vi "Top Level.vi"() -> ()   [LabVIEW 2018]
uses:
  Controls/DDS State.ctl
  <vilib>/ORNL/CSEISMIC DDS/CSEISMIC DDS Base/CSEISMIC DDS.lvclass/CSEISMIC DDS.ctl
  <vilib>/ORNL/CSEISMIC DDS/DDS Writer/Initializers/Initialize IED_Status_0 Writer.vi
  <vilib>/ORNL/CSEISMIC DDS/DDS Reader/Initializers/Initialize IED_setMicrogridID Reader.vi
  <vilib>/ORNL/CSEISMIC DDS/DDS Reader/Initializers/Initialize DER_Control Reader.vi
  <vilib>/ORNL/CSEISMIC DDS/DDS Reader/Initializers/Initialize DER_setPointP Reader.vi
  <vilib>/ORNL/CSEISMIC DDS/DDS Reader/Initializers/Initialize DER_SetPointQ Reader.vi
  <vilib>/ORNL/CSEISMIC DDS/DDS Reader/Initializers/Initialize IED_watchdogReset Reader.vi
  <vilib>/ORNL/CSEISMIC DDS/DDS Writer/Initializers/Initialize DER_Info Writer.vi
  <vilib>/ORNL/CSEISMIC DDS/DDS Writer/Initializers/Initialize DER_Measurement Writer.vi
  <vilib>/ORNL/CSEISMIC DDS/DDS Writer/Initializers/Initialize DER_Status Writer.vi
  <vilib>/ORNL/CSEISMIC DDS/DDS Writer/Initializers/Initialize IED_Status Writer.vi
  <vilib>/ORNL/CSEISMIC DDS/DDS Writer/Initializers/Initialize ES_Info Writer.vi
  <vilib>/ORNL/CSEISMIC DDS/DDS Writer/Initializers/Initialize ES_Measurement Writer.vi
  <vilib>/ORNL/CSEISMIC DDS/DDS Reader/Initializers/Initialize DER_VF Reader.vi
  <vilib>/ORNL/CSEISMIC DDS/DDS Writer/Initializers/Initialize Generator_Info Writer.vi
  <vilib>/ORNL/CSEISMIC DDS/DDS Writer/Initializers/Initialize SmartRelay_Info Writer.vi
  <vilib>/ORNL/CSEISMIC DDS/DDS Writer/Initializers/Initialize SmartRelay_Measurement Writer.vi
  <vilib>/ORNL/CSEISMIC DDS/DDS Reader/Initializers/Initialize PCC_Transition Reader.vi
  <vilib>/ORNL/CSEISMIC DDS/DDS Writer/Initializers/Initialize DER_setGenerationMode Writer.vi
  <vilib>/ORNL/CSEISMIC DDS/DDS Reader/Initializers/Initialize Relay_Control Reader.vi
  <vilib>/ORNL/CSEISMIC DDS/DDS Reader/Initializers/Initialize DER_setGenerationMode Reader.vi
  <vilib>/ORNL/CSEISMIC DDS/DDS Reader/Initializers/Initialize DER_SetPointV Reader.vi
  <vilib>/ORNL/CSEISMIC DDS/DDS Reader/Initializers/Initialize DER_SetPointF Reader.vi
  <vilib>/ORNL/CSEISMIC DDS/CSEISMIC DDS Base/Accessors/Write DDS Reference.vi
  <vilib>/ORNL/CSEISMIC DDS/DDS Reader/DDS Reader.lvclass
  C:/Program Files (x86)/National Instruments/LabVIEW 2018/vi.lib/ORNL/CSEISMIC DDS/CSEISMIC DDS Base/CSEISMIC DDS.lvclass
  <vilib>/ORNL/CSEISMIC DDS/DDS Writer/DDS Writer.lvclass
  <vilib>/ORNL/CSEISMIC DDS/DDS Reader/Initialize DDS Reader Object.vi
  <vilib>/ORNL/CSEISMIC DDS/CSEISMIC DDS Base/Error Handler.vi
  <vilib>/ORNL/CSEISMIC DDS/DDS Writer/Initialize DDS Writer Object.vi
  Global Variables/Stop (Global).vi
  Global Variables/Broadcast Topics (Global).vi
  Global Variables/Timeout Topics (Global).vi
  Global Variables/Manual Control (Global).vi
  Global Variables/DDS States (Global).vi
  Global Variables/Measurements (Global).vi
panel:
  in  "SOC":dbl=50.0
  out "PCC Closed?":bool
  in  "Manual PCC":bool=TRUE
  in  "Load P Setpoint":dbl[](array[numeric])=[50.0, 50.0, 50.0]
  in  "Timeout Gen":bool
  in  "Timeout ES2":bool
  in  "Timeout ES1":bool
  in  "Timeout PV":bool
  in  "Timeout PCC":bool
  in  "Timeout Load":bool
  in  "Broadcast Gen":bool=TRUE
  in  "Broadcast ES2":bool=TRUE
  in  "Broadcast ES1":bool=TRUE
  in  "Broadcast PV":bool=TRUE
  in  "Broadcast PCC":bool=TRUE
  in  "Broadcast Load":bool=TRUE
  out "Load DDS State":T1=enum."Shutdown"
  out "PCC DDS State":T1=enum."Shutdown"
  out "Gen DDS State":T1=enum."Shutdown"
  out "ES_2 DDS State":T1=enum."Shutdown"
  out "ES_1 DDS State":T1=enum."Shutdown"
  out "PV DDS State":T1=enum."Shutdown"
  in  "stop":bool
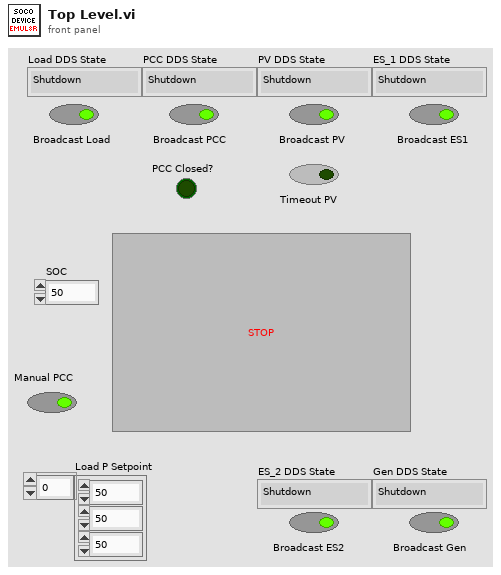
[diagram p1: front panel]
types:
  T1 = typedef "DDS State.ctl" = enum16{"Commissioning", "CheckID", "InitDDS", "ReadDDS", "WriteDDS", "CheckClose", "Close", "Shutdown"}
  T2 = typedef "Data Type DVRs.ctl" = cluster{"IED_Status":refnum<data-value>, "IED_Status_0":refnum<data-value>, "DER_Measurement":refnum<data-value>, "DER_Info":refnum<data-value>, "DER_Status":refnum<data-value>, "ES_Measurement":refnum<data-value>, "ES_Info":refnum<data-value>, "SmartRelay_Info":refnum<data-value>, "SmartRelay_Measurement":refnum<data-value>, "Meter_Info":refnum<data-value>, "Meter_Measurement":refnum<data-value>, "HVAC_Status":refnum<data-value>, "HVAC_Measurement":refnum<data-value>, "PriceData_RealTime":refnum<data-value>, "PriceData_Demand":refnum<data-value>, "PriceData_Energy":refnum<data-value>, "ForecastData_Long":refnum<data-value>, "ForecastData_Short":refnum<data-value>, "DER_Control":refnum<data-value>, "DER_SetPointP":refnum<data-value>, "DER_SetPointQ":refnum<data-value>, "DER_SetPointPF":refnum<data-value>, "DER_SetPointV":refnum<data-value>, "DER_SetPointF":refnum<data-value>, "PCC_Transition":refnum<data-value>, "DER_setGenerationMode":refnum<data-value>, "Relay_Control":refnum<data-value>, "Load_Control":refnum<data-value>, "DER_VF":refnum<data-value>, "Generator_Info":refnum<data-value>}
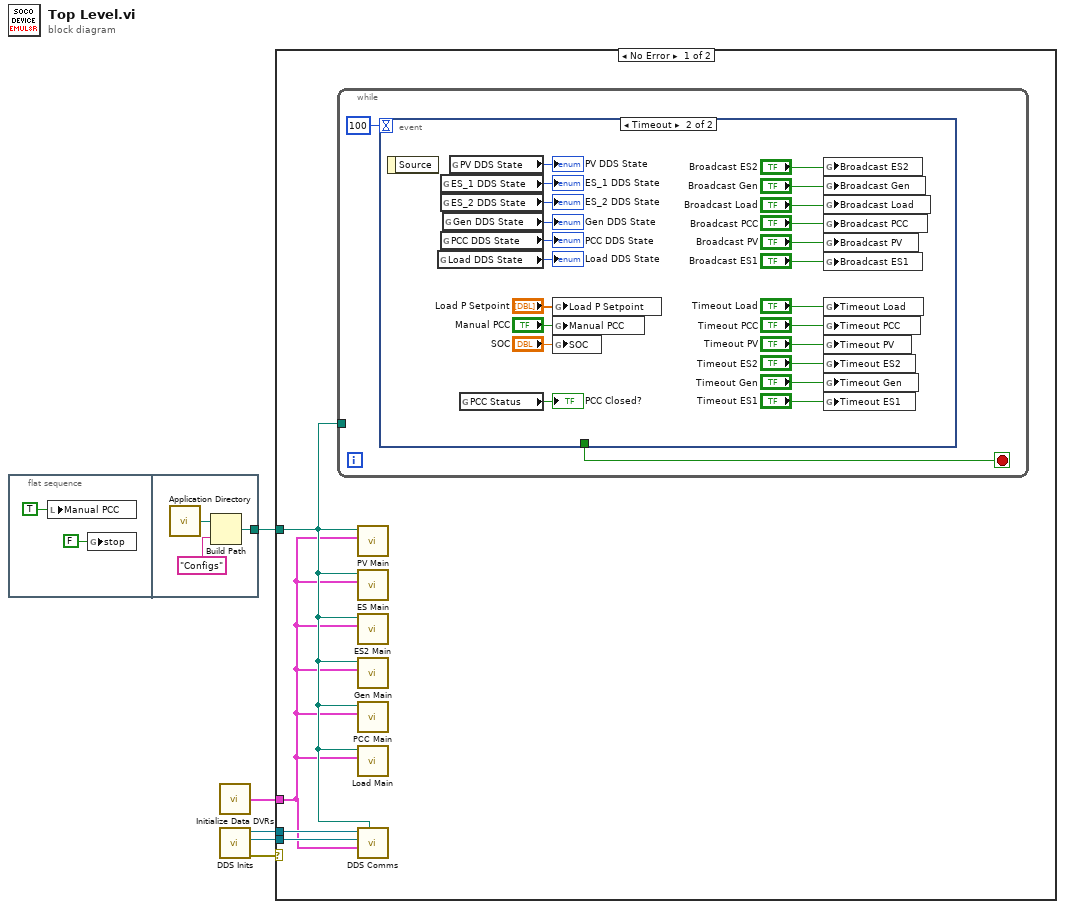
[diagram p0: block diagram]
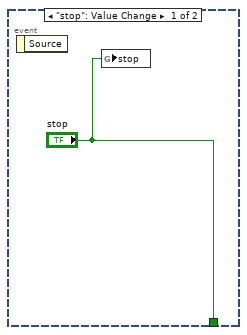
[diagram p2: hidden frame]
diagram:
  n1 = flat-sequence {
    tunnel: [w8] -> w5
    frame #0 {
      n2 = local write "Manual PCC"(TRUE ("Manual PCC")) -> ()
      n3 = global write "Stop (Global).vi" "stop"(FALSE ("stop")) -> ()
    }
    frame #1 {
      n4 = call <vilib>:"Application Directory.vi"() -> ("Application Directory"=w10:path)
      n5 = Build Path(base path=w10, name or relative path="Configs") -> (appended path=w8:path)
    }
  }
  n6 = call "Initialize Data DVRs.vi"() -> ("Data DVRs"=w1:T2)
  n7 = call "DDS Inits.vi"() -> ("error out"=w4:errorcluster, "DDS Reader out"=w2:refnum<class "DDS Reader.lvclass">, "DDS Writer out"=w3:refnum<class "DDS Writer.lvclass">)  [unwired: 9 in]
  n8 = case shown="No Error" w4 {
    tunnel: w5 -> [w12 _]
    tunnel: w3 -> [w14 _]
    tunnel: w2 -> [w13 _]
    tunnel: w1 -> [w11 _]
    frame No Error {
      n9 = while {
        tunnel: w12 -> [_]
        stop <- w16 stop-if-true
        n10 = event shown="[1] Timeout" {
          selector: _ -> [_ _]
          dyn-events: _ -> [_ _]
          timeout: 100 -> [_ _]
          tunnel: ["stop" _] -> w16
          event "stop": Value Change {
            n11 = event-data() -> ()  [unwired: 1 in, 1 out]
            n12 = global write "Stop (Global).vi" "stop"("stop") -> ()
          }
          event Timeout {
            n13 = event-data() -> ()  [unwired: 1 in, 1 out]
            n14 = global read "DDS States (Global).vi" "Load DDS State"() -> (→"Load DDS State":T1)
            n15 = global read "DDS States (Global).vi" "ES_1 DDS State"() -> (→"ES_1 DDS State":T1)
            n16 = global read "DDS States (Global).vi" "ES_2 DDS State"() -> (→"ES_2 DDS State":T1)
            n17 = global read "DDS States (Global).vi" "PCC DDS State"() -> (→"PCC DDS State":T1)
            n18 = global read "DDS States (Global).vi" "Gen DDS State"() -> (→"Gen DDS State":T1)
            n19 = global read "DDS States (Global).vi" "PV DDS State"() -> (→"PV DDS State":T1)
            n20 = global read "Measurements (Global).vi" "PCC Status"() -> (→"PCC Closed?":bool)
            n21 = global write "Manual Control (Global).vi" "Load P Setpoint"("Load P Setpoint") -> ()
            n22 = global write "Manual Control (Global).vi" "Manual PCC"("Manual PCC") -> ()
            n23 = global write "Manual Control (Global).vi" "SOC"("SOC") -> ()
            n24 = global write "Broadcast Topics (Global).vi" "Broadcast ES2"("Broadcast ES2") -> ()
            n25 = global write "Broadcast Topics (Global).vi" "Broadcast Gen"("Broadcast Gen") -> ()
            n26 = global write "Broadcast Topics (Global).vi" "Broadcast Load"("Broadcast Load") -> ()
            n27 = global write "Broadcast Topics (Global).vi" "Broadcast PCC"("Broadcast PCC") -> ()
            n28 = global write "Broadcast Topics (Global).vi" "Broadcast PV"("Broadcast PV") -> ()
            n29 = global write "Broadcast Topics (Global).vi" "Broadcast ES1"("Broadcast ES1") -> ()
            n30 = global write "Timeout Topics (Global).vi" "Timeout Load"("Timeout Load") -> ()
            n31 = global write "Timeout Topics (Global).vi" "Timeout PCC"("Timeout PCC") -> ()
            n32 = global write "Timeout Topics (Global).vi" "Timeout PV"("Timeout PV") -> ()
            n33 = global write "Timeout Topics (Global).vi" "Timeout ES2"("Timeout ES2") -> ()
            n34 = global write "Timeout Topics (Global).vi" "Timeout Gen"("Timeout Gen") -> ()
            n35 = global write "Timeout Topics (Global).vi" "Timeout ES1"("Timeout ES1") -> ()
          }
        }
      }
      n36 = call "PV Main.vi"("Data DVRs"=w11, "Config Folder"=w12) -> ()  [unwired: 10 in]
      n37 = call "ES Main.vi"("Data Type DVRs"=w11, "Config Folder"=w12) -> ()  [unwired: 10 in]
      n38 = call "ES2 Main.vi"("Data Type DVRs"=w11, "Config Folder"=w12) -> ()  [unwired: 10 in]
      n39 = call "Gen Main.vi"("Data Type DVRs"=w11, "Config Folder"=w12) -> ()  [unwired: 10 in]
      n40 = call "PCC Main.vi"("Data Type DVRs"=w11, "Config Folder"=w12) -> ()  [unwired: 10 in]
      n41 = call "Load Main.vi"("Data Type DVRs"=w11, "Config Folder"=w12) -> ()  [unwired: 10 in]
      n42 = call "DDS Comms.vi"("Config Folder"=w12, "DVR"=w11, "DDS Reader"=w13, "DDS Writer"=w14) -> ()  [unwired: 7 in, 1 out]
    }
    frame Error {
    }
  }
